vi "Read Error Queue.vi"(8 "error in (no error)":errorcluster, 11 "ErrorLog in":refnum<class "ErrorLog.lvclass">) -> (0 "error out":errorcluster, 2 "Error Queue":refnum<queue>, 3 "ErrorLog out":refnum<class "ErrorLog.lvclass">)   [LabVIEW 2019, in "ErrorLog.lvlib" / "ErrorLog.lvclass"]
uses:
  ErrorLog.lvclass
  Classes/Error/Error.lvclass
  ErrorLog.lvclass/ErrorLog.ctl
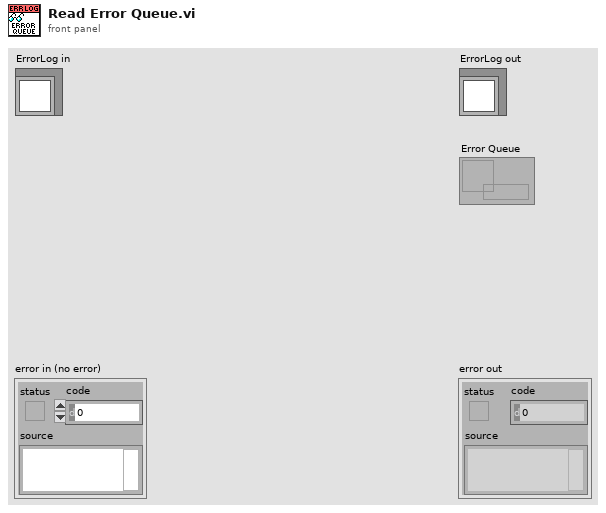
[diagram p1: front panel]
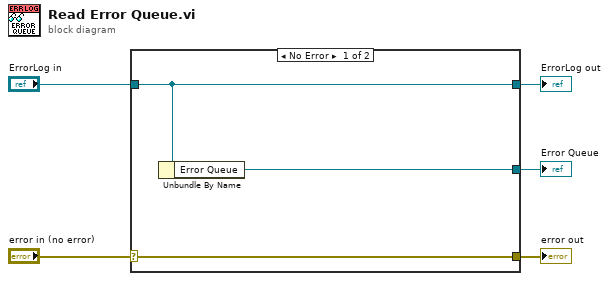
[diagram p0: block diagram]
diagram:
  n1 = case shown="No Error" "error in (no error)" {
    selector: "error in (no error)" -> [w8 w9]
    tunnel: [w8 w9] -> w4
    tunnel: [w7 w10] -> w2
    tunnel: "ErrorLog in" -> [w7 w10]
    tunnel: [w6 _] -> w1
    frame No Error {
      n2 = Unbundle By Name(w7) -> ("Error Queue"=w6:refnum<queue>)
    }
    frame Error {
    }
  }
  "error out" <- w4
  "ErrorLog out" <- w2
  "Error Queue" <- w1
